vi "fault notifications.vi"(0 "Dismiss Notification":bool, 9 "Faults":bool[](array[boolean]), 12 "Compressor Fault":bool, 13 "All Solenoid Faults":bool[](array[boolean])=[FALSE, FALSE, FALSE, FALSE, FALSE, FALSE, FALSE, FALSE], 14 "Rail Voltages":T1 {"6 volt rail"."6 volt rail voltage" format="%#_gV"; "6 volt rail"."6 volt rail current" format="%#_gA"; "5 volt rail"."5 volt rail voltage" format="%#_gV"; "5 volt rail"."5 volt rail current" format="%#_gA"; "3.3 volt rail"."3.3 volt rail voltage" format="%#_gV"; "3.3 volt rail"."3.3 volt rail current" format="%#_gA"}) -> (4 "Notification":string, 10 "Blinking?":bool, 15 "Visible?":bool)   [LabVIEW 2015]
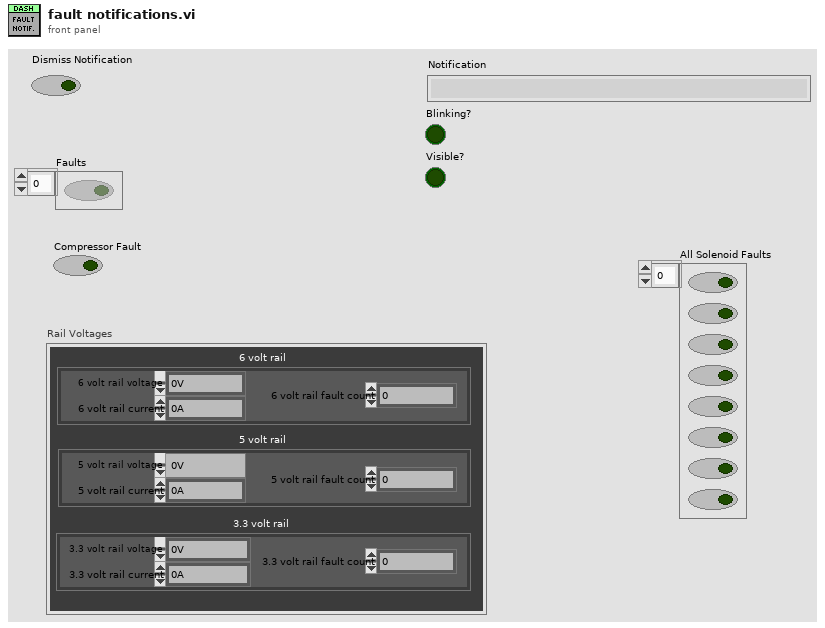
[diagram p1: front panel]
types:
  T1 = cluster{"6 volt rail":cluster{"6 volt rail voltage":dbl, "6 volt rail current":dbl, "6 volt rail fault count":dbl}, "5 volt rail":cluster{"5 volt rail voltage":dbl, "5 volt rail current":dbl, "5 volt rail fault count":dbl}, "3.3 volt rail":cluster{"3.3 volt rail voltage":dbl, "3.3 volt rail current":dbl, "3.3 volt rail fault count":dbl}}
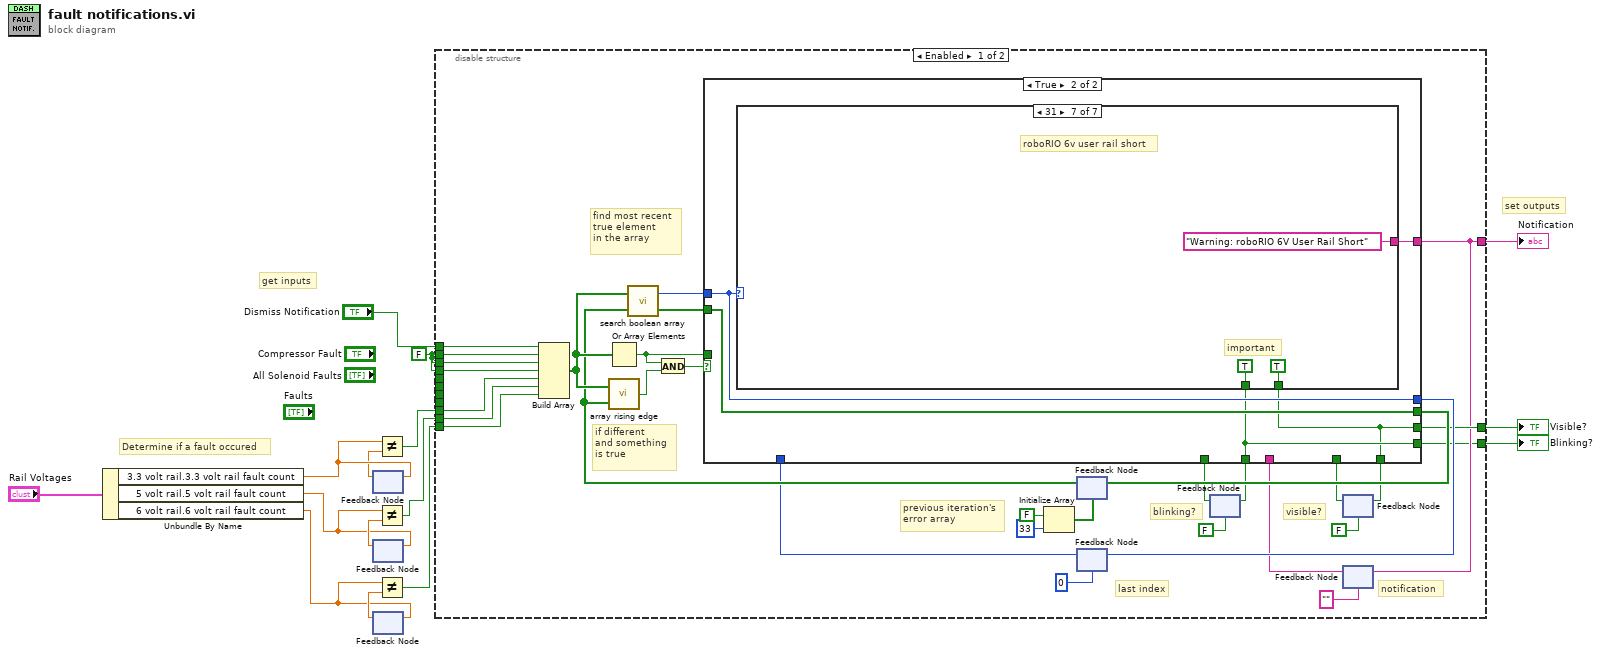
[diagram p0: block diagram]
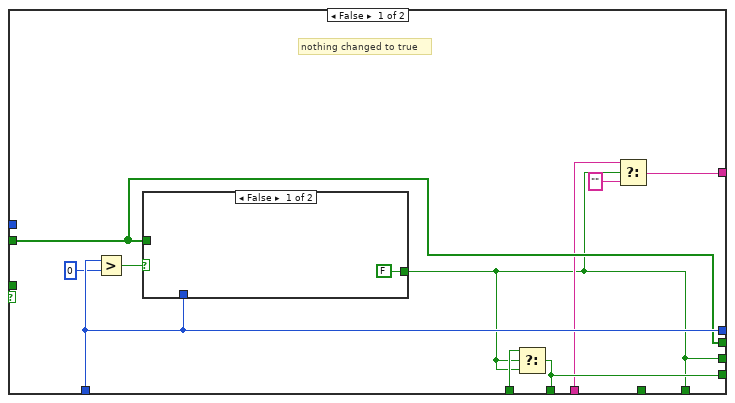
[diagram p2: hidden frame]
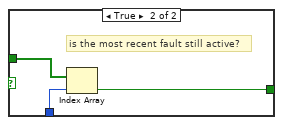
[diagram p3: hidden frame]
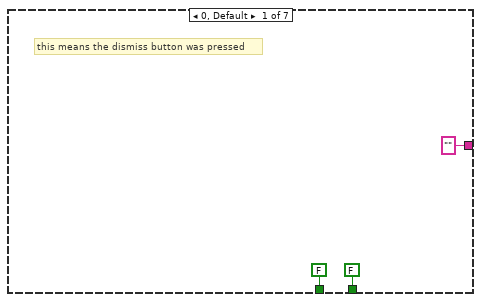
[diagram p4: hidden frame]
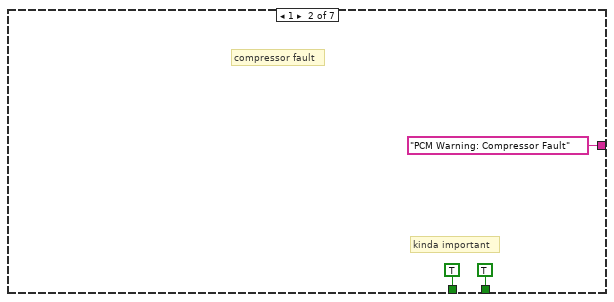
[diagram p5: hidden frame]
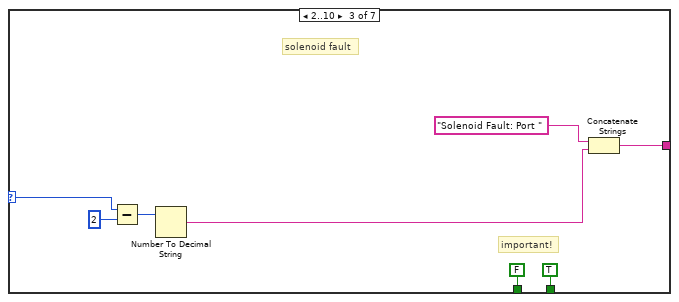
[diagram p6: hidden frame]
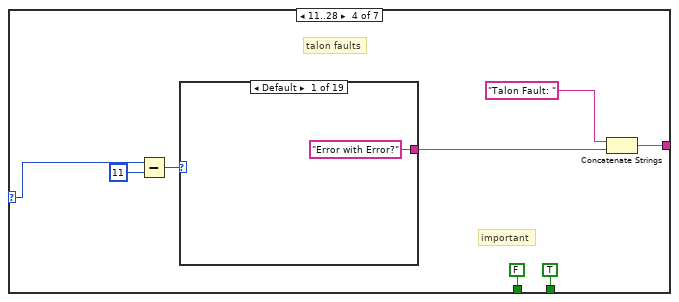
[diagram p7: hidden frame]
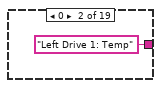
[diagram p8: hidden frame]
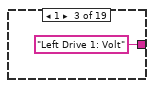
[diagram p9: hidden frame]
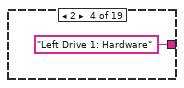
[diagram p10: hidden frame]
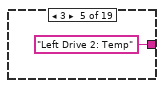
[diagram p11: hidden frame]
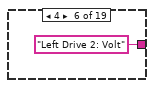
[diagram p12: hidden frame]
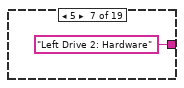
[diagram p13: hidden frame]
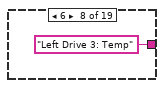
[diagram p14: hidden frame]
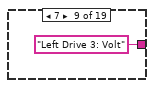
[diagram p15: hidden frame]
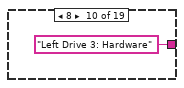
[diagram p16: hidden frame]
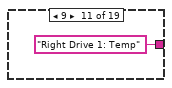
[diagram p17: hidden frame]
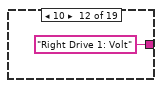
[diagram p18: hidden frame]
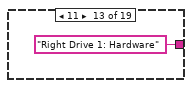
[diagram p19: hidden frame]
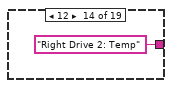
[diagram p20: hidden frame]
diagram:
  w1 = FALSE ("Compressor Fault")
  # "Determine if a fault occured"
  # "set outputs"
  # "get inputs"
  n1 = Unbundle By Name("Rail Voltages") -> ("3.3 volt rail.3.3 volt rail fault count"=w10:dbl, "5 volt rail.5 volt rail fault count"=w6:dbl, "6 volt rail.6 volt rail fault count"=w5:dbl)
  n2 = feedback #1() -> (w9:dbl)  [unwired: 1 in]
  n3 = feedback-in #1(w10) -> ()
  n4 = feedback #2() -> (w8:dbl)  [unwired: 1 in]
  n5 = feedback-in #2(w6) -> ()
  n6 = feedback #3() -> (w7:dbl)  [unwired: 1 in]
  n7 = feedback-in #3(w5) -> ()
  n8 = Not Equal?(x=w10, y=w9) -> (x != y?=w2:bool)
  n9 = Not Equal?(x=w6, y=w8) -> (x != y?=w3:bool)
  n10 = Not Equal?(x=w5, y=w7) -> (x != y?=w4:bool)
  n11 = disable-structure shown="Enabled" {
    disable-tunnel: w1 -> [w21 w152]
    disable-tunnel: w1 -> [w20 w150]
    disable-tunnel: _ -> [_ w149]
    disable-tunnel: "Dismiss Notification" -> [w47 w148]
    disable-tunnel: [w42 w143] -> w14
    disable-tunnel: _ -> [_ w142]
    disable-tunnel: _ -> [_ w141]
    disable-tunnel: _ -> [_ w140]
    disable-tunnel: w2 -> [w19 w139]
    disable-tunnel: w3 -> [w18 w138]
    disable-tunnel: w4 -> [w17 w137]
    disable-tunnel: [w35 w130] -> w13
    disable-tunnel: [w27 w122] -> w12
    disable-tunnel: w1 -> [w16 w151]
    frame Enabled {
      # "if different\nand something\nis true"
      # "find most recent\ntrue element\nin the array"
      # "notification"
      # "blinking?"
      # "previous iteration's\nerror array"
      # "last index"
      # "visible?"
      n12 = Build Array(w47, w21, w16, w20, w19, w18, w17) -> (w25:bool[])
      n13 = Or Array Elements(Boolean array=w25) -> (logical OR=w22:bool)
      n14 = Initialize Array(FALSE ("Hardware Fault"), 33 ("dimension size")) -> (w29:bool[])
      n15 = feedback #4(w29) -> (w24:bool[])
      n16 = call "array rising edge.vi"("Previous Array"=w24, "Current Array"=w25) -> ("Update Display"=w26:bool)
      n17 = call "search boolean array.vi"("Previous Array"=w24, "Array In"=w25) -> ("Array Out"=w32:bool[], "Index"=w45:i32)
      n18 = And(x=w22, y=w26) -> (x .and. y?=w28:bool)
      n19 = feedback #5(0 ("Button Pressed")) -> (w23:i32)
      n20 = feedback #6(FALSE) -> (w36:bool)
      n21 = feedback #7(FALSE) -> (w39:bool)
      n22 = feedback #8("") -> (w34:string)
      n23 = case shown="True" w28 {
        tunnel: [w52 w65] -> w46
        tunnel: w45 -> [_ w64]
        tunnel: [w55 w64] -> w44
        tunnel: w23 -> [w55 _]
        tunnel: [w49 w62] -> w42
        tunnel: [w49 w62] -> w40
        tunnel: w39 -> [_ _]
        tunnel: [w56 w63] -> w37
        tunnel: w36 -> [w57 _]
        tunnel: [w51 w66] -> w35
        tunnel: w34 -> [w50 _]
        tunnel: w32 -> [w52 w65]
        tunnel: [w56 w63] -> w27
        tunnel: w22 -> [_ _]
        frame False {
          # "nothing changed to true"
          n24 = Greater?(x=w55, y=0) -> (0:w53:bool)
          n25 = case shown="False" w53 {
            tunnel: w52 -> [_ w61]
            tunnel: w55 -> [_ w60]
            tunnel: [FALSE ("Boolean") w59] -> w49
            frame False {
            }
            frame True {
              # "is the most recent fault still active?"
              n26 = Index Array(array=w61, index=w60) -> (element=w59:bool)
            }
          }
          n27 = Select(t=w57, s=w49, f=w49) -> (s? t:f=w56:bool)
          n28 = Select(t=w50, s=w49, f="") -> (s? t:f=w51:string)
        }
        frame True {
          n29 = case shown="31" w64 {
            selector: w64 -> [_ _ w77 w82 _ _ _]
            tunnel: [FALSE TRUE FALSE FALSE TRUE TRUE TRUE] -> w63
            tunnel: ["" "PCM Warning: Compressor Fault" w74 w85 "Warning: roboRIO 3.3V User Rail Short" "Warning: roboRIO 5V User Rail Short" "Warning: roboRIO 6V User Rail Short"] -> w66
            tunnel: [FALSE TRUE TRUE TRUE TRUE TRUE TRUE] -> w62
            frame 0, Default {
              # "this means the dismiss button was pressed"
            }
            frame 1 {
              # "kinda important"
              # "compressor fault"
            }
            frame 2..10 {
              # "important!"
              # "solenoid fault"
              n30 = Subtract(x=w77, y=2) -> (x-y=w75:i32)
              n31 = Number To Decimal String(number=w75) -> (decimal integer string=w73:string)  [unwired: 1 in]
              n32 = Concatenate Strings("Solenoid Fault: Port ", w73) -> (w74:string)
            }
            frame 11..28 {
              # "important"
              # "talon faults"
              n33 = Subtract(x=w82, y=11) -> (x-y=w83:i32)
              n34 = case shown="Default" w83 {
                tunnel: ["Error with Error?" "Left Drive 1: Temp" "Left Drive 1: Volt" "Left Drive 1: Hardware" "Left Drive 2: Temp" "Left Drive 2: Volt" "Left Drive 2: Hardware" "Left Drive 3: Temp" "Left Drive 3: Volt" "Left Drive 3: Hardware" "Right Drive 1: Temp" "Right Drive 1: Volt" "Right Drive 1: Hardware" "Right Drive 2: Temp" "Right Drive 2: Volt" "Right Drive 2: Hardware" "Right Drive 3: Temp" "Right Drive 3: Volt" "Right Drive 3: Hardware"] -> w84
                frame Default {
                }
                frame 0 {
                }
                frame 1 {
                }
                frame 2 {
                }
                frame 3 {
                }
                frame 4 {
                }
                frame 5 {
                }
                frame 6 {
                }
                frame 7 {
                }
                frame 8 {
                }
                frame 9 {
                }
                frame 10 {
                }
                frame 11 {
                }
                frame 12 {
                }
                frame 13 {
                }
                frame 14 {
                }
                frame 15 {
                }
                frame 16 {
                }
                frame 17 {
                }
              }
              n35 = Concatenate Strings("Talon Fault: ", w84) -> (w85:string)
            }
            frame 29 {
              # "important"
              # "roboRIO 3.3 volt rail fault"
            }
            frame 30 {
              # "important"
              # "roboRIO 5v user rail short"
            }
            frame 31 {
              # "important"
              # "roboRIO 6v user rail short"
            }
          }
        }
      }
      n36 = feedback-in #4(w46) -> ()
      n37 = feedback-in #5(w44) -> ()
      n38 = feedback-in #6(w37) -> ()
      n39 = feedback-in #7(w40) -> ()
      n40 = feedback-in #8(w35) -> ()
    }
    frame Disabled {
      # "if different\nand something\nis true"
      # "find most recent\ntrue element\nin the array"
      # "notification"
      # "blinking?"
      # "previous iteration's\nerror array"
      # "last index"
      # "visible?"
      n41 = Build Array (concatenate)(w148, w152, w151, w150, w149, w142, w141, w140, w139, w138, w137) -> (w120:bool[])
      n42 = Or Array Elements(Boolean array=w120) -> (logical OR=w117:bool)
      n43 = Initialize Array(FALSE ("Hardware Fault"), 33 ("dimension size")) -> (w124:bool[])
      n44 = feedback #9(w124) -> (w119:bool[])
      n45 = call "array rising edge.vi"("Previous Array"=w119, "Current Array"=w120) -> ("Update Display"=w121:bool)
      n46 = call "search boolean array.vi"("Previous Array"=w119, "Array In"=w120) -> ("Array Out"=w127:bool[], "Index"=w146:i32)
      n47 = And(x=w117, y=w121) -> (x .and. y?=w123:bool)
      n48 = feedback #10(0 ("Button Pressed")) -> (w118:i32)
      n49 = feedback #11(FALSE) -> (w131:bool)
      n50 = feedback #12(FALSE) -> (w134:bool)
      n51 = feedback #13("") -> (w129:string)
      n52 = case shown="True" w123 {
        tunnel: [w157 w170] -> w147
        tunnel: w146 -> [_ w169]
        tunnel: [w160 w169] -> w145
        tunnel: w118 -> [w160 _]
        tunnel: [w154 w167] -> w143
        tunnel: [w154 w167] -> w135
        tunnel: w134 -> [_ _]
        tunnel: [w161 w168] -> w132
        tunnel: w131 -> [w162 _]
        tunnel: [w156 w171] -> w130
        tunnel: w129 -> [w155 _]
        tunnel: w127 -> [w157 w170]
        tunnel: [w161 w168] -> w122
        tunnel: w117 -> [_ _]
        frame False {
          # "nothing changed to true"
          n53 = Greater?(x=w160, y=0) -> (0:w158:bool)
          n54 = case shown="False" w158 {
            tunnel: w157 -> [_ w166]
            tunnel: w160 -> [_ w165]
            tunnel: [FALSE ("Boolean") w164] -> w154
            frame False {
            }
            frame True {
              # "is the most recent fault still active?"
              n55 = Index Array(array=w166, index=w165) -> (element=w164:bool)
            }
          }
          n56 = Select(t=w162, s=w154, f=w154) -> (s? t:f=w161:bool)
          n57 = Select(t=w155, s=w154, f="") -> (s? t:f=w156:string)
        }
        frame True {
          n58 = case shown="21..28" w169 {
            selector: w169 -> [_ w177 _ _ _ _ w199 _ _ _ _]
            tunnel: [FALSE FALSE TRUE TRUE TRUE FALSE FALSE TRUE TRUE TRUE TRUE] -> w168
            tunnel: ["" w179 "PDP Warning: Battery Voltage Fault" "PDP Warning: Temperature Fault" "PDP Warning: Hardware Fault" "PDP Warning: Compressor Fault" w197 "DANGER: roboRIO Input Voltage Brown Out" "Warning: roboRIO 3.3V User Rail Short" "Warning: roboRIO 5V User Rail Short" "Warning: roboRIO 6V User Rail Short"] -> w171
            tunnel: [FALSE TRUE TRUE TRUE TRUE TRUE TRUE TRUE TRUE TRUE TRUE] -> w167
            frame 0, Default {
              # "this means the dismiss button was pressed"
            }
            frame 1..16 {
              # "not super important"
              # "Indexes 1-16 for PDP channels 0-15"
              # "Faults from PDP"
              n59 = Decrement(x=w177) -> (x-1=w178:i32)
              n60 = Number To Decimal String(number=w178, width (-)=i16 0) -> (decimal integer string=w180:string)
              n61 = Concatenate Strings("PDP Current Fault: Channel ", w180) -> (w179:string)
            }
            frame 17 {
              # "kinda important"
              # "battery voltage fault"
            }
            frame 18 {
              # "important!"
              # "temperature fault"
            }
            frame 19 {
              # "important"
              # "(hardware problem)"
              # "hardware fault"
            }
            frame 20 {
              # "not super important"
              # "compressor fault"
            }
            frame 21..28 {
              # "not super important"
              # "indexes 21-28"
              # "solenoids 0-7"
              # "solenoid faults"
              n62 = Subtract(x=w199, y=21) -> (x-y=w200:i32)
              n63 = Number To Decimal String(number=w200, width (-)=i16 0) -> (decimal integer string=w201:string)
              n64 = Concatenate Strings("PCM Current Fault: Solenoid ", w201) -> (w197:string)
            }
            frame 29 {
              # "important"
              # "roboRIO input voltage brown out"
            }
            frame 30 {
              # "important"
              # "roboRIO 3.3v user rail short"
            }
            frame 31 {
              # "important"
              # "roboRIO 5v user rail short"
            }
            frame 32 {
              # "important"
              # "roboRIO 6v user rail short"
            }
          }
        }
      }
      n65 = feedback-in #9(w147) -> ()
      n66 = feedback-in #10(w145) -> ()
      n67 = feedback-in #11(w132) -> ()
      n68 = feedback-in #12(w135) -> ()
      n69 = feedback-in #13(w130) -> ()
    }
  }
  "Notification" <- w13
  "Visible?" <- w14
  "Blinking?" <- w12
